vi "CH_LM Config Backlight.vi"(0 "Meter Index":i32, 1 "AC Auto Off (Off)":bool, 2 "AC Auto Off Timer (1 min)":i32=1, 3 "Battery Auto Off (Off)":bool, 4 "Battery Auto Off Timer (1 min)":i32=1, 5 "error in (no error)":errorcluster, 6 "State (On)":bool=TRUE, 7 "Timeout / ms (3000)":i32=3000, 8 "Action (query)":bool, 9 "Lock Timeout / ms (1000)":i32=1000) -> (11 "Lock timed out":bool, 12 "State":bool, 14 "Meter Index":i32, 15 "AC Auto Off":bool, 16 "AC Auto Off Timer / min":i32, 17 "Battery Auto Off":bool, 18 "Battery Auto Off Timer / min":i32, 19 "error out":errorcluster)   [LabVIEW 2012, in "CH_LM.lvlib"]
doc: "This VI will query and set parameters pertinent to the backlight.\n\nThe meter can be configured to automatically turn off the backlight after the specified front panel idle period."
uses:
  CH_LM.lvlib
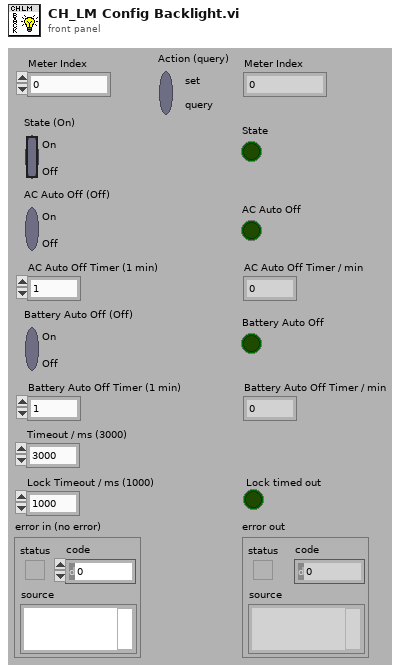
[diagram p1: front panel]
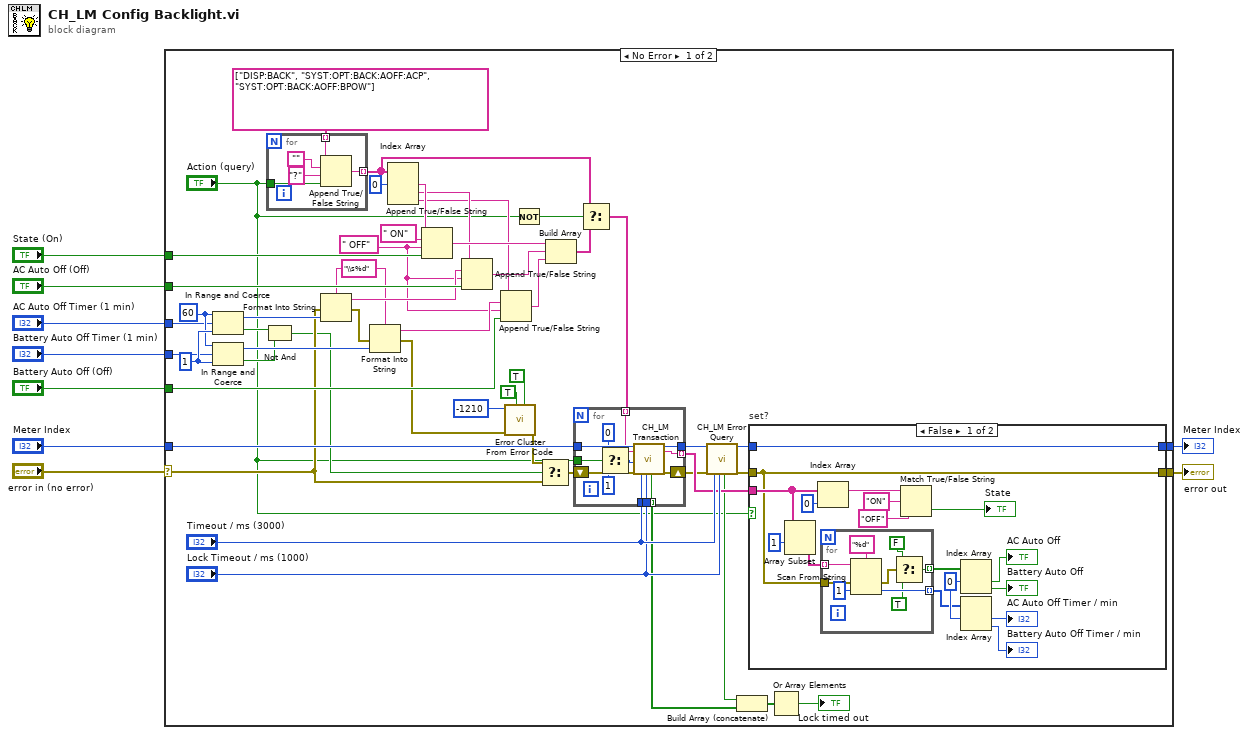
[diagram p0: block diagram]
diagram:
  n1 = case shown="No Error" "error in (no error)" {
    selector: "error in (no error)" -> [w18 w109]
    tunnel: [w60 w109] -> w9
    tunnel: "Meter Index" -> [w61 w108]
    tunnel: [w59 w108] -> w6
    tunnel: "Battery Auto Off Timer (1 min)" -> [w50 _]
    tunnel: "AC Auto Off Timer (1 min)" -> [w51 _]
    tunnel: "AC Auto Off (Off)" -> [w54 _]
    tunnel: "State (On)" -> [w53 _]
    tunnel: "Battery Auto Off (Off)" -> [w52 _]
    frame No Error {
      w31 = "\\s%d" ("format string")
      w25 = " OFF" ("false string")
      w56 = 1 ("lower limit")
      w55 = 60 ("upper limit")
      n2 = In Range and Coerce(upper limit=w55, x=w51, lower limit=w56) -> (coerced(x)=w49:i32, In Range?=w17:bool)
      n3 = In Range and Coerce(upper limit=w55, x=w50, lower limit=w56) -> (coerced(x)=w48:i32, In Range?=w16:bool)
      n4 = Not And(1:w16, 2:w17) -> (0:w15:bool)
      n5 = for {
        tunnel: "Action (query)" -> [w64]
        tunnel: [w63] -> w12 mode=indexing
        tunnel: string[] ["DISP:BACK", "SYST:OPT:BACK:AOFF:ACP", "SYST:OPT:BACK:AOFF:BPOW"] -> [w62] mode=indexing
        n6 = Append True/False String(1:w64, 2:"?" ("true string"), 3:"", 4:w62) -> (0:w63:string)
      }
      n7 = Format Into String(format string=w31, error in=w18, w49) -> (resulting string=w32:string, error out=w27:errorcluster)  [unwired: 1 in]
      n8 = Format Into String(format string=w31, error in=w27, w48) -> (resulting string=w26:string, error out=w21:errorcluster)  [unwired: 1 in]
      n9 = Index Array(array=w12, index #1=0 ("index")) -> (element #1=w35:string, element #2=w33:string, element #3=w29:string)  [unwired: 2 in]
      n10 = Append True/False String(1:w53, 2:w25, 3:" ON" ("true string"), 4:w35) -> (0:w34:string)
      n11 = Append True/False String(1:w54, 2:w25, 3:w32, 4:w33) -> (0:w30:string)
      n12 = Append True/False String(1:w52, 2:w25, 3:w26, 4:w29) -> (0:w28:string)
      n13 = call <vilib>:"Error Cluster From Error Code.vi"("is warning? (False)"=TRUE, "show call chain? (False)"=TRUE, "error in (no error)"=w21, "error code (0)"=-1210) -> ("error out"=w20:errorcluster)  [unwired: 5 out]
      n14 = Not(x="Action (query)") -> (.not. x?=w13:bool)
      n15 = Select(t=w20, s=w15, f=w18) -> (s? t:f=w19:errorcluster)
      n16 = Build Array(w34, w30, w28) -> (w11:string[])
      n17 = Select(t=w12, s=w13, f=w11) -> (s? t:f=w10:string[])
      n18 = for {
        tunnel: w61 -> [w78]
        tunnel: [w77] -> w47 mode=indexing
        tunnel: [w73] -> w46
        tunnel: [w71] -> w41 mode=indexing
        tunnel: "Timeout / ms (3000)" -> [w70]
        tunnel: "Lock Timeout / ms (1000)" -> [w69]
        tunnel: "Action (query)" -> [w68]
        tunnel: w10 -> [w67] mode=indexing
        shift-right: [w72] -> w44
        shift-left: w19 -> [w79]
        n19 = Select(t=0, s=w68, f=1 ("NofStrings (-1:all)")) -> (s? t:f=w75:i32)
        n20 = call "CH_LM Transaction.vi"("Meter Index"=w78, "Command String"=w67, "NofStrings (-1:all)"=w75, "error in (no error)"=w79, "Timeout / ms (3000)"=w70, "Lock Timeout / ms (1000)"=w69) -> ("Lock timed out"=w71:bool, "Meter Index"=w73:i32, "Response"=w77:string, "error out"=w72:errorcluster)  [unwired: 10 out]
      }
      n21 = call "CH_LM Error Query.vi"("Meter Index"=w46, "error in (no error)"=w44, "Timeout / ms (3000)"="Timeout / ms (3000)", "Lock Timeout / ms (1000)"="Lock Timeout / ms (1000)") -> ("Lock timed out"=w42:bool, "Meter Index"=w45:i32, "error out"=w43:errorcluster)  [unwired: 13 out]
      n22 = Build Array (concatenate)(w42, w41) -> (w40:bool[])
      n23 = case "set?" shown="False" "Action (query)" {
        tunnel: w47 -> [w90 _]
        tunnel: w43 -> [w87 w107]
        tunnel: [w87 w107] -> w60
        tunnel: w45 -> [w96 w106]
        tunnel: [w96 w106] -> w59
        frame False {
          w85 = 0 ("index")
          n24 = Array Subset(array=w90, index=1) -> (w88:string[])  [unwired: 1 in]
          n25 = Index Array(array=w90, index=0) -> (element=w95:string)
          n26 = for {
            tunnel: w88 -> [w105] mode=indexing
            tunnel: w87 -> [w104]
            tunnel: [w102] -> w84 mode=indexing
            tunnel: [w98] -> w86 mode=indexing
            n27 = Scan From String(format string="%d", input string=w105, error in=w104, default 1=1 ("default value 1")) -> (error out=w101:errorcluster, output 1=w102:i32)  [unwired: 1 in, 2 out]
            n28 = Select(t=FALSE, s=w101, f=TRUE) -> (s? t:f=w98:bool)
          }
          n29 = Match True/False String(2:"OFF" ("false string"), 3:"ON" ("true string"), 4:w95) -> (0:→"State":bool)  [unwired: 1 out]
          n30 = Index Array(array=w86, index #1=w85) -> (element #1=→"AC Auto Off":bool, element #2=→"Battery Auto Off":bool)  [unwired: 1 in]
          n31 = Index Array(array=w84, index #1=w85) -> (element #1=→"AC Auto Off Timer / min":i32, element #2=→"Battery Auto Off Timer / min":i32)  [unwired: 1 in]
        }
        frame True {
        }
      }
      n32 = Or Array Elements(Boolean array=w40) -> (logical OR=→"Lock timed out":bool)
    }
    frame Error {
    }
  }
  "error out" <- w9
  "Meter Index" <- w6
